vi "String.Date to Variables.vi"() -> (3 "Variable List":string[][](array[string]))   [LabVIEW 2018]
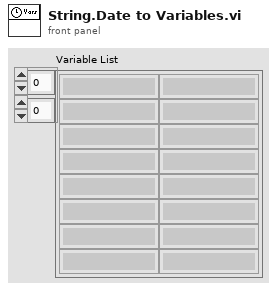
[diagram p1: front panel]
types:
  T1 = typedef "LVDateTimeRec.ctl" = cluster{"fractional second":dbl, "second":i32, "minute":i32, "hour":i32, "day of month":i32, "month":i32, "year":i32, "day of week":i32, "day of year":i32, "DST":i32}
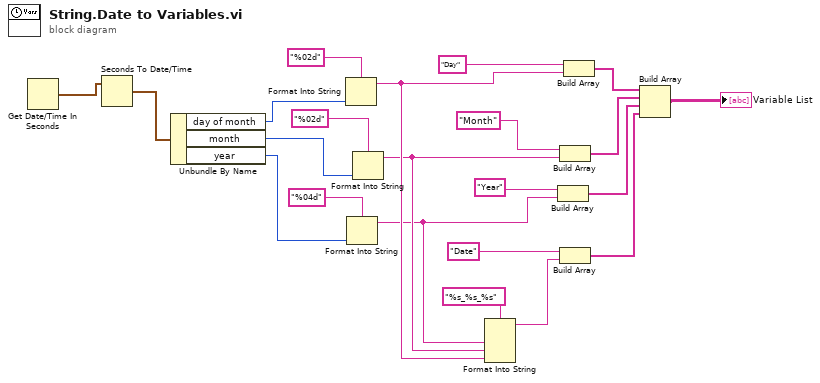
[diagram p0: block diagram]
diagram:
  n1 = Get Date/Time In Seconds() -> (seconds since 1Jan1904=w22:timestamp)
  n2 = Seconds To Date/Time(time stamp (now)=w22) -> (date time rec=w21:T1)  [unwired: 1 in]
  n3 = Unbundle By Name(w21) -> ("day of month"=w20:i32, "month"=w19:i32, "year"=w18:i32)
  n4 = Format Into String(format string="%02d", w20) -> (resulting string=w5:string)  [unwired: 2 in, 1 out]
  n5 = Format Into String(format string="%04d", w18) -> (resulting string=w3:string)  [unwired: 2 in, 1 out]
  n6 = Format Into String(format string="%02d", w19) -> (resulting string=w4:string)  [unwired: 2 in, 1 out]
  n7 = Format Into String(format string="%s_%s_%s", w3, w4, w5) -> (resulting string=w2:string)  [unwired: 2 in, 1 out]
  n8 = Build Array("Year", w3) -> (w8:string[])
  n9 = Build Array("Month", w4) -> (w9:string[])
  n10 = Build Array("Date", w2) -> (w7:string[])
  n11 = Build Array("Day", w5) -> (w10:string[])
  n12 = Build Array(w10, w9, w8, w7) -> (→"Variable List":string[][])
